vi "Get Path to svn.vi"() -> (3 "working directory":path=path "C:/Program Files/CollabNet/Subversion Client")   [LabVIEW 2015]
uses:
  <vilib>/Utility/config.llb/NI_LVConfig.lvlib
  <vilib>/Utility/config.llb/Read Key (Path).vi
  <vilib>/Utility/config.llb/Write Key (Path).vi
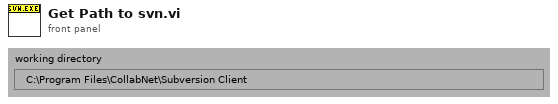
[diagram p1: front panel]
types:
  T1 = typedef "NI_LVConfig.lvlib/Config Data RefNum.ctl" = refnum<k1>
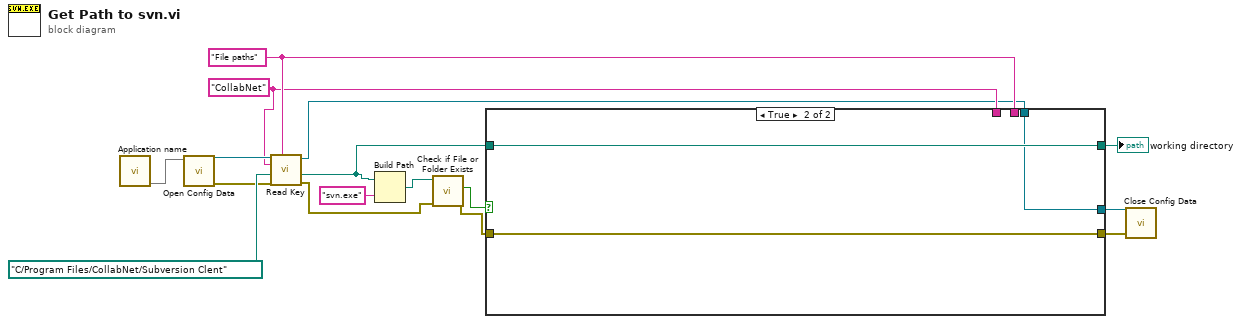
[diagram p0: block diagram]
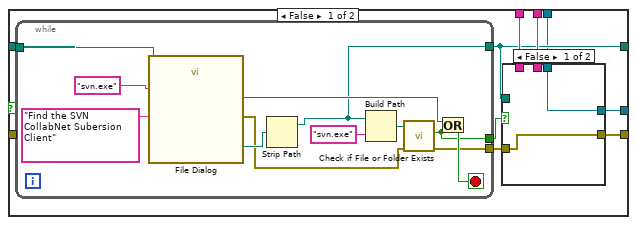
[diagram p2: hidden frame]
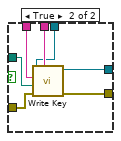
[diagram p3: hidden frame]
diagram:
  w6 = "File paths" ("section")
  w5 = "CollabNet" ("key")
  n1 = call "Application name.vi"() -> (0:w16)  [unwired: 4 in, 3 out]
  n2 = call <vilib>:"Open Config Data.vi"("configuration file path"=w16) -> ("error out"=w10:errorcluster, "refnum"=w15:T1)  [unwired: 8 in, 1 out]
  n3 = call-poly <vilib>:"Read Key.vi"("section"=w6, "error in (no error)"=w10, "default value"=path "C:/Program Files/CollabNet/Subversion Clent" ("working directory"), "key"=w5, "refnum"=w15) -> ("error out"=w11:errorcluster, "value"=w7:path, "refnum out"=w4:T1)  [unwired: 3 in, 1 out]
  n4 = Build Path(base path=w7, name or relative path="svn.exe") -> (appended path=w12:path)
  n5 = call <vilib>:"Check if File or Folder Exists.vi"("error in (no error)"=w11, "path"=w12) -> ("error out"=w1:errorcluster, "file or folder exists?"=w9:bool)  [unwired: 7 in, 1 out]
  n6 = case shown="True" w9 {
    tunnel: [w21 w49] -> w8
    tunnel: w7 -> [w25 w49]
    tunnel: w6 -> [w24 _]
    tunnel: w5 -> [w23 _]
    tunnel: w4 -> [w20 w48]
    tunnel: [w18 w47] -> w3
    tunnel: [w17 w48] -> w2
    tunnel: w1 -> [_ w47]
    frame False {
      n7 = while {
        tunnel: w25 -> [w46]
        tunnel: [w37] -> w21
        tunnel: [w36] -> w22
        tunnel: [w35] -> w19
        stop <- w38 stop-if-true
        n8 = call "File Dialog"("start path"=w46, "prompt"="Find the SVN CollabNet Subersion Client", "pattern (all files)"="svn.exe" ("pattern label")) -> ("selected path"=w41:path, "cancelled"=w39:bool, "error out"=w40:errorcluster)  [unwired: 9 in, 1 out]
        n9 = Strip Path(path=w41) -> (stripped path=w37:path)  [unwired: 1 out]
        n10 = Build Path(base path=w37, name or relative path="svn.exe") -> (appended path=w43:path)
        n11 = call <vilib>:"Check if File or Folder Exists.vi"("error in (no error)"=w40, "path"=w43) -> ("error out"=w35:errorcluster, "file or folder exists?"=w36:bool)  [unwired: 7 in, 1 out]
        n12 = Or(x=w39, y=w36) -> (x .or. y?=w38:bool)
      }
      n13 = case shown="False" w22 {
        tunnel: w24 -> [_ w34]
        tunnel: w23 -> [_ w33]
        tunnel: w21 -> [_ w32]
        tunnel: w20 -> [w27 w31]
        tunnel: w19 -> [w26 w30]
        tunnel: [w26 w29] -> w18
        tunnel: [w27 w28] -> w17
        frame False {
        }
        frame True {
          n14 = call-poly <vilib>:"Write Key.vi"("section"=w34, "error in (no error)"=w30, "value"=w32, "key"=w33, "refnum"=w31) -> ("error out"=w29:errorcluster, "refnum out"=w28:T1)  [unwired: 4 in, 1 out]
        }
      }
    }
    frame True {
    }
  }
  "working directory" <- w8
  n15 = call <vilib>:"Close Config Data.vi"("error in (no error)"=w3, "refnum"=w2) -> ()  [unwired: 8 in, 2 out]
